vi "generateIntegers.vi"(6 "timeout (10000)":i32=10000, 8 "error in (no error)":errorcluster, 11 "Parameters":T2={"params"={"apiKey"="", "n"=0, "min"=0, "max"=0, "replacement"=TRUE, "base"=10}, "id"=0.0} {"params"."base" items=["2"=2, "8"=8, "10"=10, "16"=16]}) -> (0 "error out":errorcluster, 3 "Response":T1, 4 "error data":string[](array[string]))   [LabVIEW 2014, in "Random JSON API.lvlib"]
uses:
  Random JSON API.lvlib
  Type Defs/generateIntegersRequest.ctl
  Type Defs/generateIntegersResponse.ctl
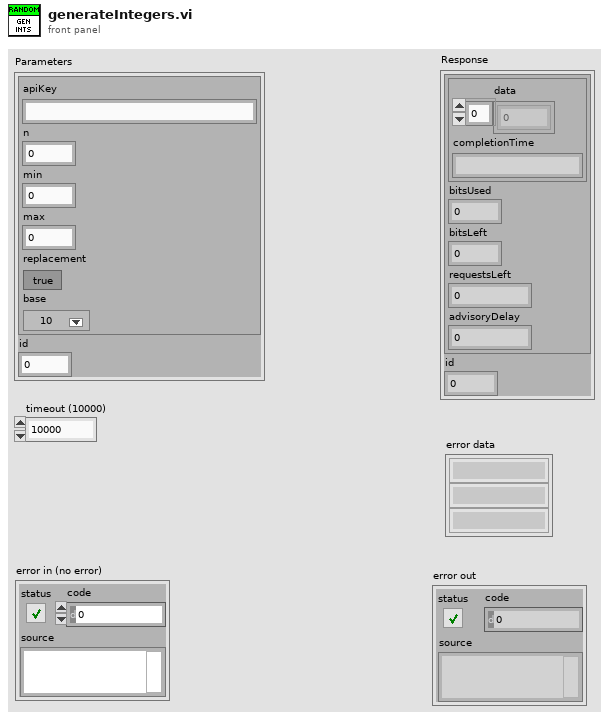
[diagram p1: front panel]
types:
  T1 = typedef "Random JSON API.lvlib/generateIntegersResponse.ctl" = cluster{"result":cluster{"random":cluster{"data":i32[], "completionTime":string}, "bitsUsed":i32, "bitsLeft":i32, "requestsLeft":i32, "advisoryDelay":i32}, "id":dbl}
  T2 = typedef "Random JSON API.lvlib/generateIntegersRequest.ctl" = cluster{"params":cluster{"apiKey":string, "n":i32, "min":i32, "max":i32, "replacement":bool, "base":i32}, "id":dbl}
  T3 = cluster{"apiKey":string, "n":i32, "min":i32, "max":i32, "replacement":bool, "base":i32}
  T4 = cluster{"jsonrpc":string, "method":string, "params":cluster{"apiKey":string, "n":i32, "min":i32, "max":i32, "replacement":bool, "base":i32}, "id":dbl}
  T5 = cluster{"completionTime":string, "bitsUsed":i32, "bitsLeft":i32, "requestsLeft":i32, "advisoryDelay":i32}
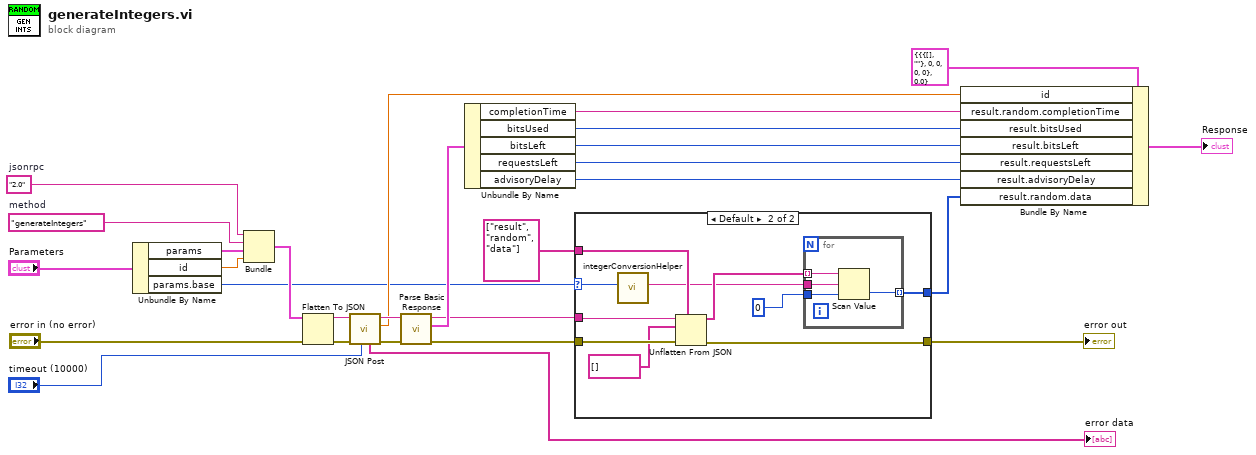
[diagram p0: block diagram]
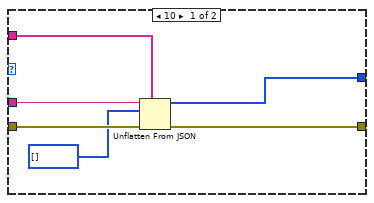
[diagram p2: hidden frame]
diagram:
  w24 = "generateIntegers"  # method
  w25 = "2.0"  # jsonrpc
  n1 = Unbundle By Name("Parameters") -> ("params"=w18:T3, "id"=w17:dbl, "params.base"=w1:i32)
  n2 = Bundle("jsonrpc"=w25, "method"=w24, "params"=w18, "id"=w17) -> (w23:T4)  [unwired: 1 in]
  n3 = Flatten To JSON(anything=w23, error in (no error)="error in (no error)") -> (JSON string=w19:string, 11:w20:errorcluster)  [unwired: 1 in]
  n4 = call "JSON Post.vi"("timeout (10000)"="timeout (10000)", "error in (no error)"=w20, "Request JSON String"=w19) -> ("error out"=w27:errorcluster, "id"=w15:dbl, "Response JSON String"=w16:string, "error data"=→"error data":string[])  [unwired: 5 in]
  n5 = call "Parse Basic Response.vi"("error in (no error)"=w27, "body in"=w16) -> ("error out"=w8:errorcluster, "result cluster"=w14:T5, "body out"=w7:string)  [unwired: 7 in]
  n6 = Unbundle By Name(w14) -> ("completionTime"=w13:string, "bitsUsed"=w12:i32, "bitsLeft"=w11:i32, "requestsLeft"=w10:i32, "advisoryDelay"=w9:i32)
  n7 = case shown="Default" w1 {
    selector: w1 -> [_ w40]
    tunnel: w8 -> [w34 w44]
    tunnel: [w33 w37] -> w26
    tunnel: [w31 w39] -> w6
    tunnel: w7 -> [w32 w42]
    tunnel: string[] ["result", "random", "data"] ("path") -> [w29 w41]
    frame 10 {
      n8 = Unflatten From JSON(path=w29, JSON string=w32, type and defaults=i32[] [], error in (no error)=w34) -> (value=w31:i32[], error out=w33:errorcluster)  [unwired: 3 in]
    }
    frame Default {
      n9 = call "integerConversionHelper.vi"("base"=w40) -> ("base conversion string"=w35:string)  [unwired: 10 in]
      n10 = Unflatten From JSON(path=w41, JSON string=w42, type and defaults=string[] [], error in (no error)=w44) -> (value=w36:string[], error out=w37:errorcluster)  [unwired: 3 in]
      n11 = for {
        tunnel: [w48] -> w39 mode=indexing
        tunnel: w36 -> [w47] mode=indexing
        tunnel: w35 -> [w45]
        tunnel: 0 -> [w46]
        n12 = Scan Value(string=w47, format string=w45, default (0 dbl)=w46) -> (value=w48:i32)  [unwired: 1 out]
      }
    }
  }
  "error out" <- w26
  n13 = Bundle By Name(cluster=T1 {"result"={"random"={"data"=[], "completionTime"=""}, "bitsUsed"=0, "bitsLeft"=0, "requestsLeft"=0, "advisoryDelay"=0}, "id"=0.0} ("Response"), "id"=w15, "result.random.completionTime"=w13, "result.bitsUsed"=w12, "result.bitsLeft"=w11, "result.requestsLeft"=w10, "result.advisoryDelay"=w9, "result.random.data"=w6) -> (→"Response":T1)
